vi "Set Sample Rate And Start.vi"(7 "AI?":bool, 8 "error in":errorcluster, 9 "Indices":i32[](array[numeric]), 10 "Rate":dbl, 11 "task in":refnum<k21>) -> (0 "error out":errorcluster, 3 "task out":refnum<k21>)   [LabVIEW 2014, in "DAQmx Module Runtime.lvclass"]
uses:
  DAQmx Module Runtime.lvclass
  <vilib>/DAQmx/configure/timing.llb/DAQmx Timing (Sample Clock).vi
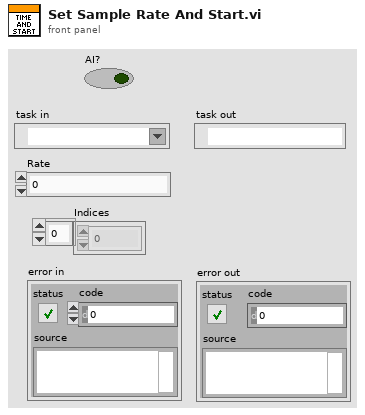
[diagram p1: front panel]
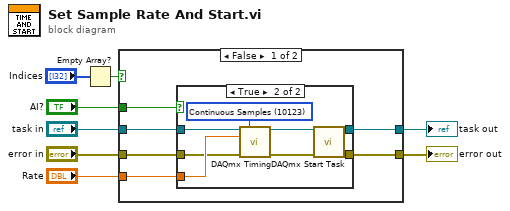
[diagram p0: block diagram]
diagram:
  n1 = Empty Array?(array="Indices") -> (empty?=w1:bool)
  n2 = case shown="False" w1 {
    tunnel: "Rate" -> [w14 _]
    tunnel: [w13 w26] -> w7
    tunnel: [w12 w25] -> w6
    tunnel: "error in" -> [w11 w25]
    tunnel: "task in" -> [w10 w26]
    tunnel: "AI?" -> [w9 _]
    frame False {
      n3 = case shown="True" w9 {
        tunnel: w14 -> [_ w23]
        tunnel: w10 -> [w16 w22]
        tunnel: w11 -> [w15 w21]
        tunnel: [w16 w18] -> w13
        tunnel: [w15 w17] -> w12
        frame False {
        }
        frame True {
          w24 = 10123 items=["Finite Samples"=10178, "Continuous Samples"=10123, "Hardware Timed Single Point"=12522] ("sample mode")
          n4 = call-poly <vilib>:"DAQmx Timing.vi"("task/channels in"=w22, "sample mode"=w24, "rate"=w23, "error in"=w21) -> ("task out"=w20:refnum<k21>, "error out"=w19:errorcluster)  [unwired: 10 in]
          n5 = call <vilib>:"DAQmx Start Task.vi"("task/channels in"=w20, "error in"=w19) -> ("task out"=w18:refnum<k21>, "error out"=w17:errorcluster)  [unwired: 12 in]
        }
      }
    }
    frame True {
    }
  }
  "task out" <- w7
  "error out" <- w6
